vi "Remove Row.vi"(8 "error in":errorcluster, 11 "MulticolumnListbox in":refnum<vi>) -> (0 "error out":errorcluster)   [LabVIEW 2017, in "DTacq Plot Display Library.lvlib"]
uses:
  DTacq Plot Display Library.lvlib
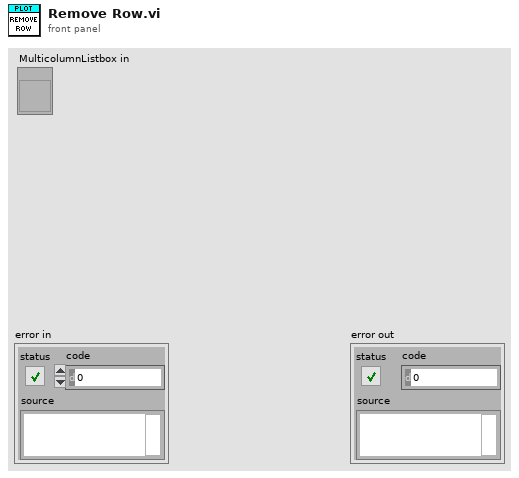
[diagram p1: front panel]
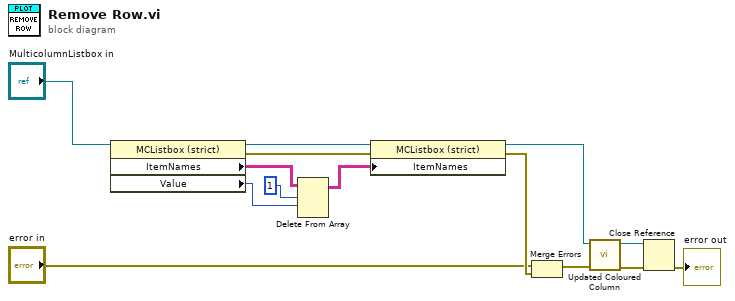
[diagram p0: block diagram]
diagram:
  n1 = property class="MCListbox (strict)"(reference="MulticolumnListbox in") -> (reference out=w12:refnum<vi>, error out=w13:errorcluster, "ItemNames"=w8:string[][], "Value"=w9:i32)  [unwired: 1 in]
  n2 = Delete From Array(array=w8, length=1, index (row)=w9) -> (array with subset deleted=w11:string[][])  [unwired: 1 in, 1 out]
  n3 = property class="MCListbox (strict)"(reference=w12, error in=w13, "ItemNames"=w11) -> (reference out=w14:refnum<vi>, error out=w6:errorcluster)
  n4 = Merge Errors("error in", w6) -> (w4:errorcluster)
  n5 = call "Updated Coloured Column.vi"("error in"=w4, "MulticolumnListbox in"=w14) -> ("error out"=w3:errorcluster, "MulticolumnListbox Out"=w2:refnum<vi>)  [unwired: 8 in]
  n6 = Close Reference(reference=w2, error in (no error)=w3) -> (error out=→"error out":errorcluster)
